vi "AOout.vi"(8 "错误输入（无错误）":errorcluster, 9 "波形参数":cluster{"波形类型":u16, "幅值":dbl, "频率":dbl}[](array[cluster])=[{"波形类型"=0, "幅值"=1.0, "频率"=10.0}] {"频率" format="%0.2p"; "幅值" format="%0.2p"; "波形类型" items=["正弦波", "三角波", "方波", "锯齿波"]}, 10 "Hardware Configuration":T2 caption="硬件配置", 11 "队列输入":refnum<queue>) -> (0 "错误输出":errorcluster, 1 "数值":i32, 2 "波形图":waveform(dbl)[](graph)=[{"t0"=timestamp(0 s since 1904-01-01), "dt"=0.001, "Y"=[]}], 3 "Hardware Resources out":T1={"Max Input"=0.0, "Min Input"=0.0, "Sample Rate"=0.0, "Sample Num"=0.0, "DAQmx Task"="", "物理通道"="Dev1/ao0"}, 5 "Message":string caption="消息")   [LabVIEW 2014]
uses:
  Hardware Configures.ctl
  support/Message Queue/Message Cluster.ctl
  controls/State.ctl
  support/Message Queue/Enqueue Message (Single).vi
  support/Message Queue/Message Queue.lvlib
  HardWareConfig.lvlib
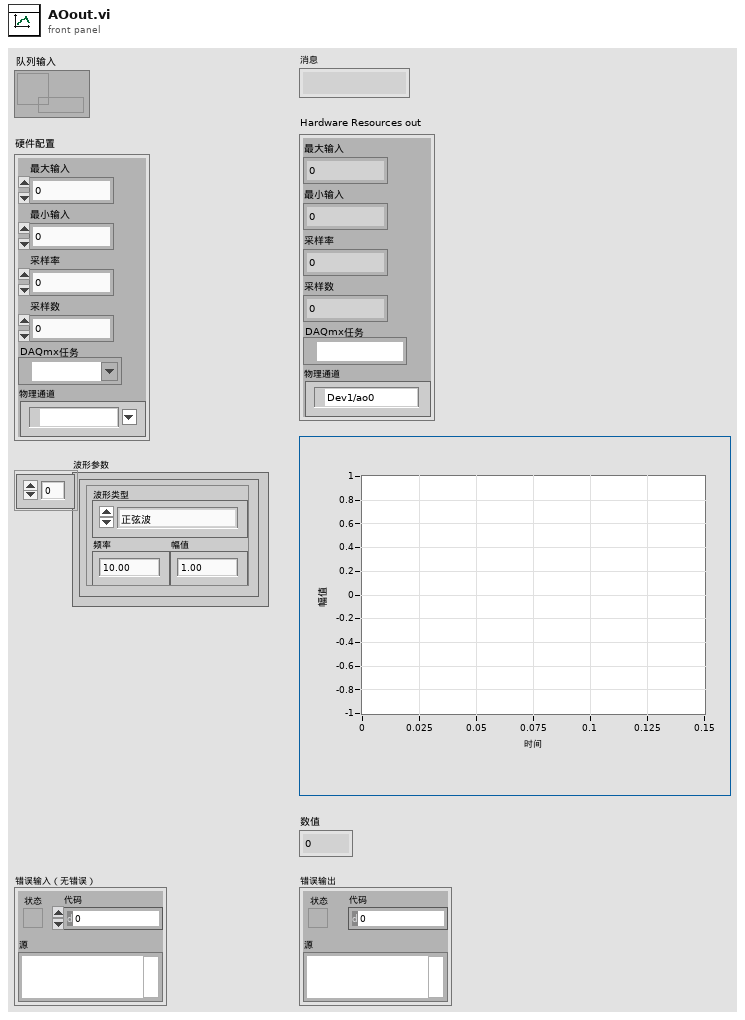
[diagram p1: front panel]
types:
  T1 = typedef "HardWareConfig.lvlib/Hardware Configures.ctl" = cluster{"Max Input":dbl, "Min Input":dbl, "Sample Rate":dbl, "Sample Num":dbl, "DAQmx Task":refnum<k21>, "物理通道":tag}
  T2 = cluster{"Max Input":dbl, "Min Input":dbl, "Sample Rate":dbl, "Sample Num":dbl, "DAQmx Task":refnum<k21>, "物理通道":tag}
  T3 = typedef "State.ctl" = enum16{"Idle", "AOoutputting"}
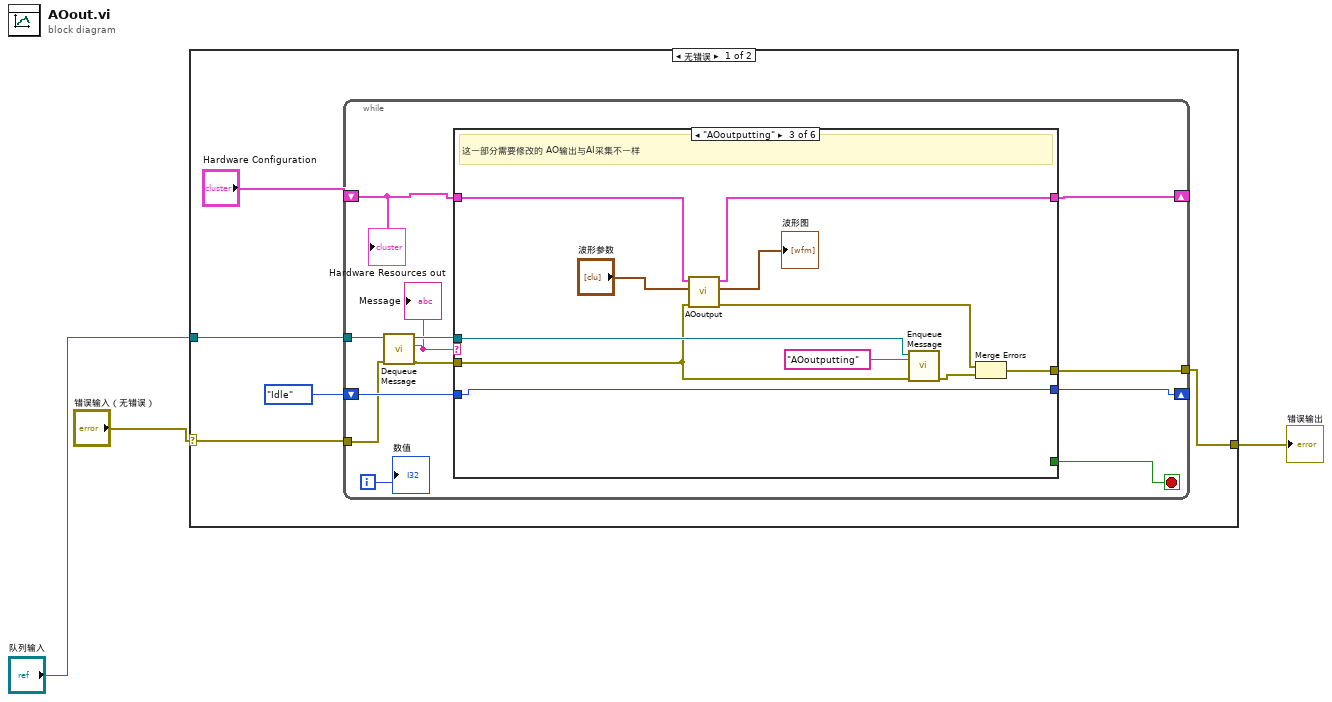
[diagram p0: block diagram]
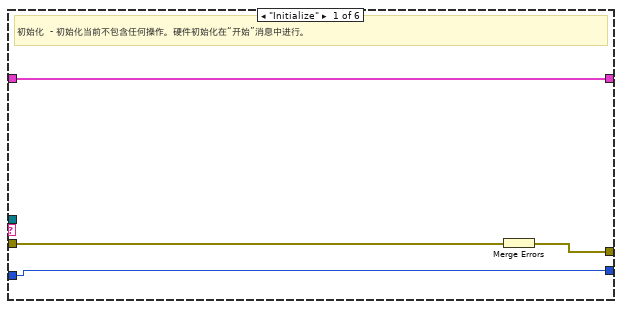
[diagram p2: hidden frame]
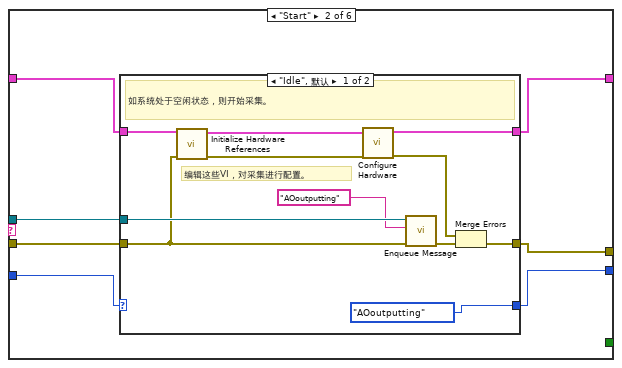
[diagram p3: hidden frame]
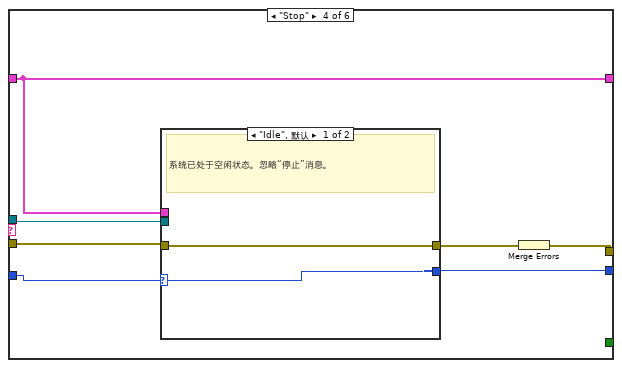
[diagram p5: hidden frame]
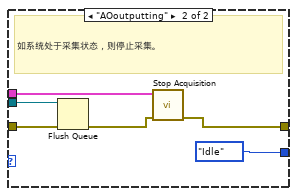
[diagram p6: hidden frame]
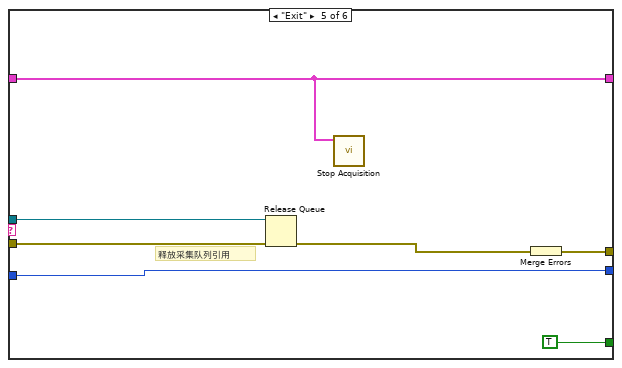
[diagram p7: hidden frame]
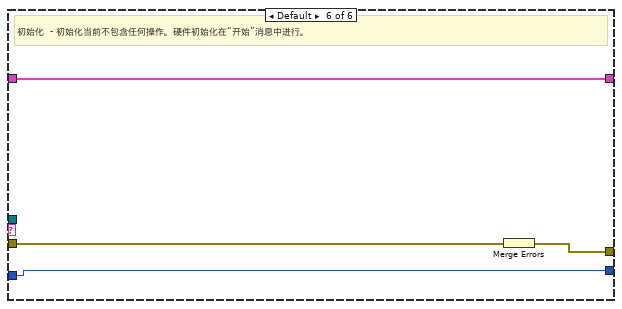
[diagram p8: hidden frame]
diagram:
  n1 = case shown="无错误" "错误输入（无错误）" {
    selector: "错误输入（无错误）" -> [w7 w83]
    tunnel: [w8 w83] -> w2
    tunnel: "队列输入" -> [w4 _]
    frame No Error {
      n2 = while {
        tunnel: [w20] -> w8
        tunnel: w7 -> [w11]
        shift-right: [w17] -> _
        shift-left: State."Idle" ("State") -> [w16]
        shift-right: [w18] -> _
        shift-left: "Hardware Configuration" -> [w19]
        tunnel: w4 -> [w9]
        i -> [w10]
        stop <- w15 stop-if-true
        n3 = call "Dequeue Message.vi"("error in (no error)"=w11, "Message Queue"=w9) -> ("error out"=w13:errorcluster, "Message"=w12:string, "dup Message Queue"=w14:refnum<queue>)  [unwired: 6 in, 1 out]
        "Message" <- w12
        n4 = case shown="\"AOoutputting\"" w12 {
          tunnel: [w22 w26 w53 w59 w74 w80] -> w20
          tunnel: w19 -> [w24 w27 w56 w57 w72 w82]
          tunnel: [w24 w25 w55 w57 w72 w82] -> w18
          tunnel: w13 -> [w23 w29 w50 w63 w77 w81]
          tunnel: [w21 w30 w46 w60 w76 w79] -> w17
          tunnel: w16 -> [w21 w31 w46 w61 w76 w79]
          tunnel: w14 -> [_ w28 w51 w62 w78 _]
          tunnel: [_ _ _ _ TRUE _] -> w15
          frame "Initialize" {
            # "初始化  - 初始化当前不包含任何操作。硬件初始化在“开始”消息中进行。"
            n5 = Merge Errors(w23) -> (w22:errorcluster)
          }
          frame "Start" {
            n6 = case shown="\"Idle\", 默认" w31 {
              selector: w31 -> [_ w43]
              tunnel: [w42 w45] -> w26
              tunnel: w27 -> [w36 w44]
              tunnel: w29 -> [w35 w45]
              tunnel: w28 -> [w40 _]
              tunnel: [w32 w44] -> w25
              tunnel: [State."AOoutputting" ("State") w43] -> w30
              frame "Idle", Default {
                # "编辑这些VI，对采集进行配置。"
                # "如系统处于空闲状态，则开始采集。"
                n7 = call "Initialize Hardware References.vi"("error in (no error)"=w35, "Hardware Resources in"=w36) -> ("error out"=w34:errorcluster, "Hardware Resources out"=w33:T1)  [unwired: 8 in]
                n8 = call "Configure Hardware.vi"("error in (no error)"=w34, "Hardware Resources in"=w33) -> ("error out"=w39:errorcluster, "Hardware Resources out"=w32:T1)  [unwired: 8 in]
                n9 = call-poly "Enqueue Message.vi"("error in (no error)"=w35, "Message"="AOoutputting", "Message Queue"=w40) -> ("error out"=w41:errorcluster)  [unwired: 7 in, 1 out]
                n10 = Merge Errors(w39, w41) -> (w42:errorcluster)
              }
              frame "AOoutputting" {
                # "系统已开始采集。忽略“开始”消息。"
              }
            }
          }
          frame "AOoutputting" {
            # "这一部分需要修改的 AO输出与AI采集不一样"
            n11 = call "AOoutput.vi"("error in (no error)"=w50, "波形参数"="波形参数", "Hardware Resources in"=w56) -> ("error out"=w54:errorcluster, "波形图"=→"波形图":waveform(dbl)[], "Hardware Resources out"=w55:T1)  [unwired: 6 in]
            n12 = call-poly "Enqueue Message.vi"("error in (no error)"=w50, "Message"="AOoutputting", "Message Queue"=w51) -> ("error out"=w49:errorcluster)  [unwired: 7 in, 1 out]
            n13 = Merge Errors(w54, w49) -> (w53:errorcluster)
          }
          frame "Stop" {
            n14 = case shown="\"Idle\", 默认" w61 {
              selector: w61 -> [w65 _]
              tunnel: w63 -> [w64 w71]
              tunnel: w62 -> [_ w70]
              tunnel: [w65 State."Idle" ("State")] -> w60
              tunnel: [w64 w66] -> w58
              tunnel: w57 -> [_ w68]
              frame "Idle", Default {
                # "系统已处于空闲状态。忽略“停止”消息。"
              }
              frame "AOoutputting" {
                # "如系统处于采集状态，则停止采集。"
                n15 = Flush Queue(queue=w70, error in (no error)=w71) -> (error out=w67:errorcluster)  [unwired: 2 out]
                n16 = call "Stop Acquisition.vi"("error in (no error)"=w67, "Hardware Resources in"=w68) -> ("error out"=w66:errorcluster)  [unwired: 9 in]
              }
            }
            n17 = Merge Errors(w58) -> (w59:errorcluster)
          }
          frame "Exit" {
            # "释放采集队列引用"
            n18 = Release Queue(queue=w78, error in (no error)=w77) -> (error out=w73:errorcluster)  [unwired: 1 in, 2 out]
            n19 = call "Stop Acquisition.vi"("Hardware Resources in"=w72) -> ()  [unwired: 10 in, 1 out]
            n20 = Merge Errors(w73) -> (w74:errorcluster)
          }
          frame Default {
            # "初始化  - 初始化当前不包含任何操作。硬件初始化在“开始”消息中进行。"
            n21 = Merge Errors(w81) -> (w80:errorcluster)
          }
        }
        "数值" <- w10
        "Hardware Resources out" <- w19
      }
    }
    frame Error {
    }
  }
  "错误输出" <- w2
